vi "Facade.vi"(0 "Data In":T4, 2 "Display State In":T2, 3 "Container State":T3) -> (6 "Data Out":T4, 7 "Display State Out":T2, 8 "Action":T1)   [LabVIEW 2015, in "Pulse Train.xctl"]
uses:
  Pulse Train.xctl
  Data.vi
  Classes/Waveforms/Pulse Train/Pulse Train.lvclass
  <vilib>/_xctls/Container State.ctl
  State.vi
  <vilib>/_xctls/Action.ctl
  Classes/Waveforms/Pulse Train/Pulse Train.lvclass/Pulse Train.ctl
  Classes/Waveforms/Pulse Train/Read Shape.vi
  Classes/Waveforms/Pulse Train/Read Width (us).vi
  Classes/Waveforms/Pulse Train/Read Rate (Hz).vi
  Classes/Waveforms/Pulse Train/Write Shape.vi
  Classes/Waveforms/Pulse Train/Write Width (us).vi
  Classes/Waveforms/Pulse Train/Write Rate (Hz).vi
  <vilib>/_xctls/XControlSupport.lvlib
panel:
  in  "Rate (Hz)":dbl
  in  "Width (us)":string
  in  "Shape":string
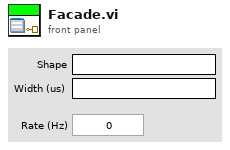
[diagram p1: front panel]
types:
  T1 = typedef "XControlSupport.lvlib/Action.ctl" = cluster{"Data Changed?":bool, "State Changed?":bool, "Action Name":string}
  T2 = typedef "Pulse Train.xctl/State.vi" = cluster{"Numeric":dbl}
  T3 = typedef "XControlSupport.lvlib/Container State.ctl" = cluster{"Indicator?":bool, "Run Mode?":bool, " Refnum":refnum<vi>}
  T4 = typedef "Pulse Train.xctl/Data.vi" = refnum<class "Pulse Train.lvclass">
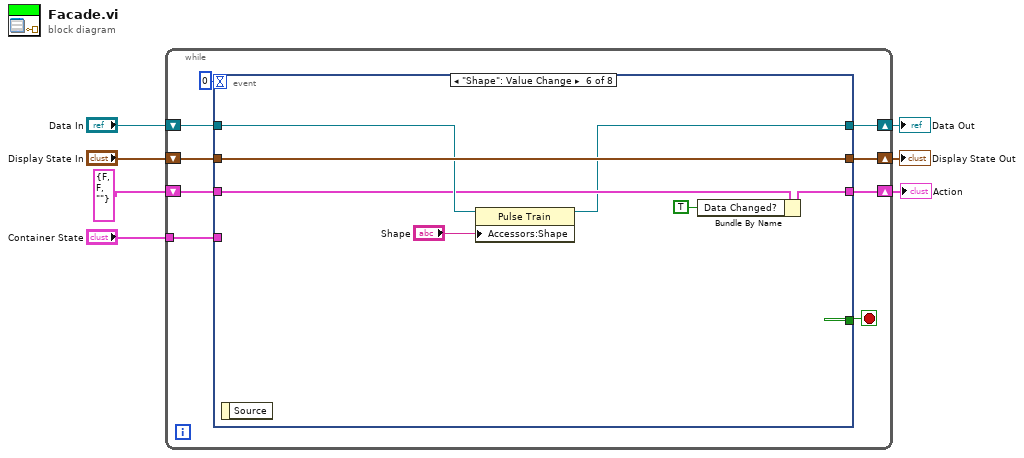
[diagram p0: block diagram]
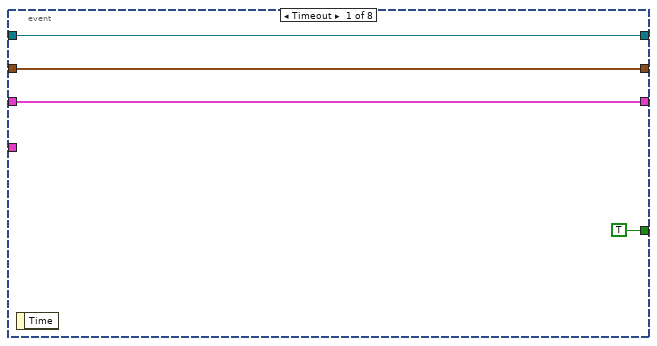
[diagram p2: hidden frame]
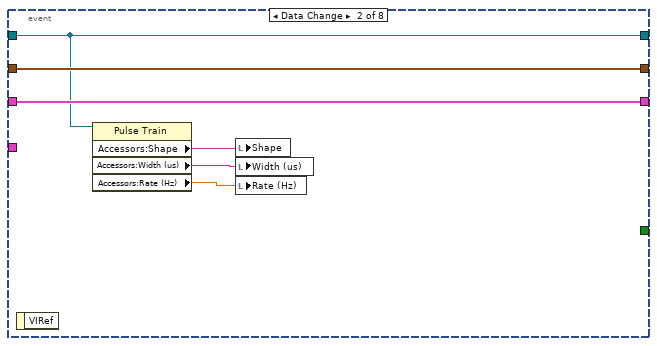
[diagram p3: hidden frame]
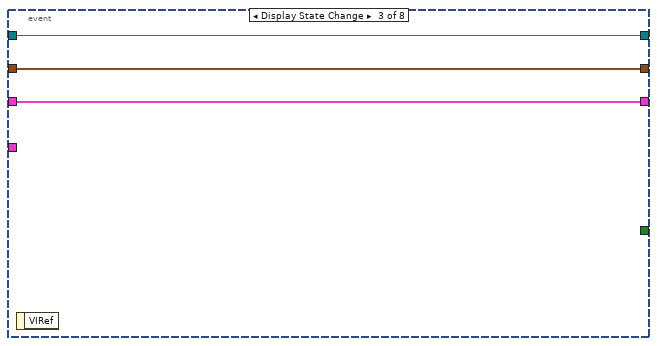
[diagram p4: hidden frame]
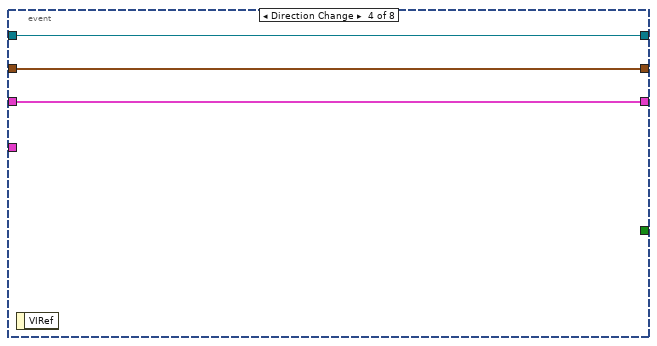
[diagram p5: hidden frame]
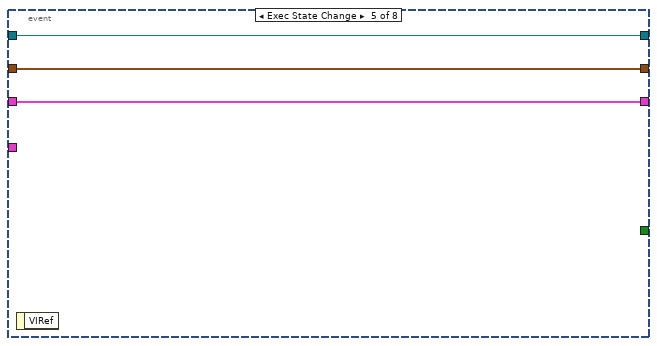
[diagram p6: hidden frame]
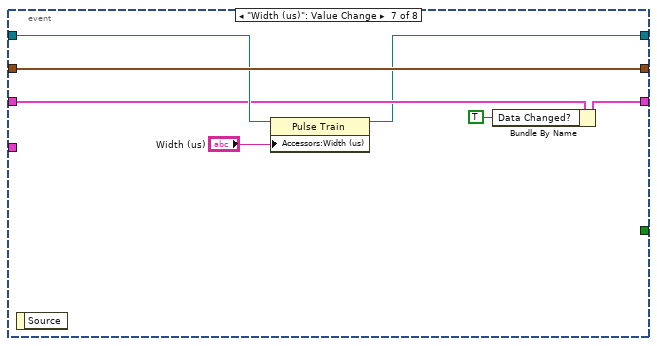
[diagram p7: hidden frame]
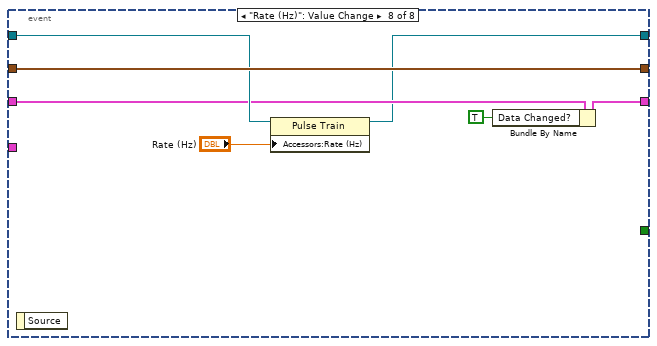
[diagram p8: hidden frame]
diagram:
  n1 = while {
    shift-right: [w15] -> w4
    shift-left: "Display State In" -> [w16]
    tunnel: "Container State" -> [w12]
    shift-right: [w10] -> w7
    shift-left: "Data In" -> [w11]
    shift-right: [w8] -> w2
    shift-left: T1 {"Data Changed?"=FALSE, "State Changed?"=FALSE, "Action Name"=""} ("Action") -> [w9]
    stop <- w14 stop-if-true
    n2 = event shown="[5] \"Shape\": Value Change" {
      selector: _ -> [_ _ _ _ _ _ _ _]
      dyn-events: _ -> [_ _ _ _ _ _ _ _]
      timeout: 0 -> [_ _ _ _ _ _ _ _]
      tunnel: w16 -> [w18 w26 w29 w32 w35 w42 w49 w56]
      tunnel: [w18 w26 w29 w32 w35 w42 w49 w56] -> w15
      tunnel: [TRUE _ _ _ _ _ _ _] -> w14
      tunnel: w12 -> [_ _ _ _ _ _ _ _]
      tunnel: w11 -> [w17 w24 w28 w31 w34 w41 w48 w55]
      tunnel: [w17 w24 w28 w31 w34 w39 w46 w53] -> w10
      tunnel: [w19 w25 w27 w30 w33 w38 w45 w52] -> w8
      tunnel: w9 -> [w19 w25 w27 w30 w33 w40 w47 w54]
      event Timeout {
        n3 = event-data() -> ()  [unwired: 1 in, 1 out]
      }
      event Data Change {
        n4 = event-data() -> ()  [unwired: 1 in, 1 out]
        n5 = property class="Pulse Train"(reference=w24) -> ("Accessors:Shape"=w23:string, "Accessors:Width (us)"=w22:string, "Accessors:Rate (Hz)"=w21:dbl)  [unwired: 1 in, 2 out]
        n6 = local write "Shape"(w23) -> ()
        n7 = local write "Width (us)"(w22) -> ()
        n8 = local write "Rate (Hz)"(w21) -> ()
      }
      event Display State Change {
        n9 = event-data() -> ()  [unwired: 1 in, 1 out]
      }
      event Direction Change {
        n10 = event-data() -> ()  [unwired: 1 in, 1 out]
      }
      event Exec State Change {
        n11 = event-data() -> ()  [unwired: 1 in, 1 out]
      }
      event "Shape": Value Change {
        n12 = event-data() -> ()  [unwired: 1 in, 1 out]
        n13 = property class="Pulse Train"(reference=w41, "Accessors:Shape"="Shape") -> (reference out=w39:T4)  [unwired: 1 in, 1 out]
        n14 = Bundle By Name(cluster=w40, "Data Changed?"=TRUE) -> (w38:T1)
      }
      event "Width (us)": Value Change {
        n15 = event-data() -> ()  [unwired: 1 in, 1 out]
        n16 = property class="Pulse Train"(reference=w48, "Accessors:Width (us)"="Width (us)") -> (reference out=w46:T4)  [unwired: 1 in, 1 out]
        n17 = Bundle By Name(cluster=w47, "Data Changed?"=TRUE) -> (w45:T1)
      }
      event "Rate (Hz)": Value Change {
        n18 = event-data() -> ()  [unwired: 1 in, 1 out]
        n19 = property class="Pulse Train"(reference=w55, "Accessors:Rate (Hz)"="Rate (Hz)") -> (reference out=w53:T4)  [unwired: 1 in, 1 out]
        n20 = Bundle By Name(cluster=w54, "Data Changed?"=TRUE) -> (w52:T1)
      }
    }
  }
  "Display State Out" <- w4
  "Data Out" <- w7
  "Action" <- w2
